vi "parse bmp.vi"(8 "error in (no error)":errorcluster, 11 "<bmp> string":string) -> (0 "error out":errorcluster, 3 "bmp data":T1)   [LabVIEW 2018, in "Data Parser.lvclass"]
uses:
  Data Parser.lvclass
  Bmp data.ctl
panel:
  out "debug array":string[](array[string])
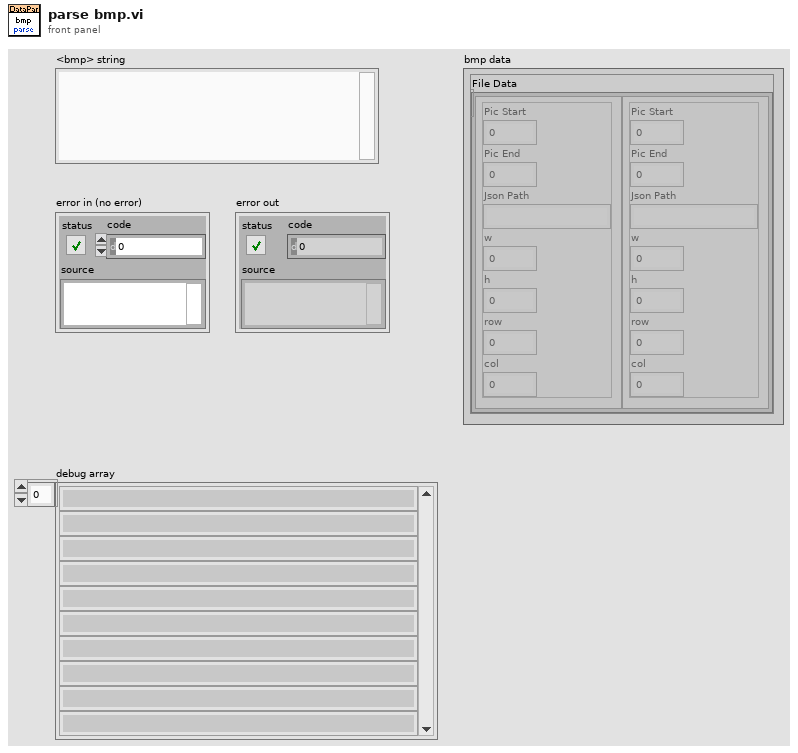
[diagram p1: front panel]
types:
  T1 = typedef "Data Parser.lvclass/Bmp data.ctl" = cluster{"File Data":cluster{"Pic Start":i32, "Pic End":i32, "Json Path":string, "w":i32, "h":i32, "row":i32, "col":i32}[]}
  T2 = cluster{"pic start":i32, "pic end":i32, "json path":string, "w":i32, "h":i32, "row":i32, "col":i32}
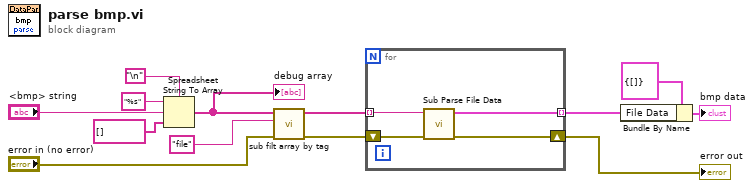
[diagram p0: block diagram]
diagram:
  n1 = Spreadsheet String To Array(delimiter (Tab)="\n", format string="%s", spreadsheet string="<bmp> string", array type (2D Dbl)=string[] []) -> (array=w9:string[])
  "debug array" <- w9
  n2 = call "sub filt array by tag.vi"("error in"="error in (no error)", "tag"="file" ("String"), "string array"=w9) -> ("error out"=w2:errorcluster, "filted string array"=w7:string[])  [unwired: 7 in]
  n3 = for {
    tunnel: [w17] -> w5 mode=indexing
    tunnel: w7 -> [w16] mode=indexing
    shift-right: [w14] -> w1
    shift-left: w2 -> [w15]
    n4 = call "Sub Parse File Data.vi"("error in (no error)"=w15, "input string"=w16) -> ("error out"=w14:errorcluster, "file data"=w17:T2)  [unwired: 8 in]
  }
  "error out" <- w1
  n5 = Bundle By Name(cluster=T1 {"File Data"=[]} ("bmp data"), "File Data"=w5) -> (→"bmp data":T1)
